vi "Charge Calibration_2011.vi"(0 "Screen&Camera 2":T1={"Screen Orientation"="Regular", "Screen angle"="Flat", "Lens"=enum."FL1-f8x08", "Calibration (mm/pix)"=1.0}, 1 "ROI infos":T3={"npix-X"=512, "npix-Y"=384, "Left [pix]"=0.0, "Top [pix]"=0.0}, 2 "Image (Counts)":dbl[][](array[numeric]), 3 "Filters":cluster{"Name":string, "#Filters":dbl}[](array[cluster])=[{"Name"="BG38", "#Filters"=0.0}, {"Name"="F40", "#Filters"=0.0}, {"Name"="F70", "#Filters"=0.0}, {"Name"="oldBP", "#Filters"=0.0}], 4 "Electron energy (MeV)":dbl=100.0) -> (7 "Image (pC)":dbl[][](array[numeric]))   [LabVIEW 2020]
uses:
  SubVis/ScreenCam2_TypDEf.ctl
  MagAnalysis_Online_Bella/SubVis/CamAndObj_TypDEf.ctl
panel:
  # "Screen Charge calibration\n10/06/10 - Guillaume Plateau"
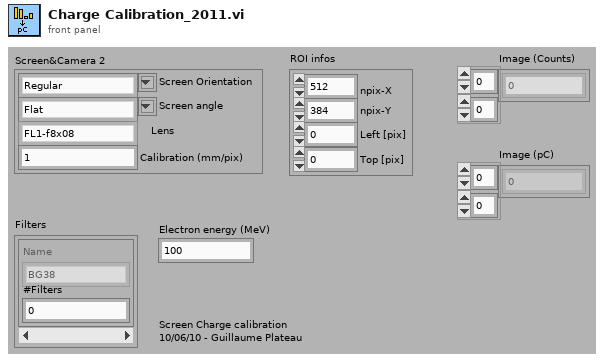
[diagram p1: front panel]
types:
  T1 = typedef "ScreenCam2_TypDEf.ctl" = cluster{"Screen Orientation":string, "Screen angle":string, "Lens":T2, "Calibration (mm/pix)":dbl}
  T2 = typedef "CamAndObj_TypDEf.ctl" = enum16{"FL1-f8x08", "FL1-f8x06", "FL1-f8", "ch300-f50", "FL2G-f8", "FL3M14-f8", "FL3M14-f8x08", "FL3M14-f8x08(2x2)", "aca720-f8", "aca1440-f8"}
  T3 = cluster{"npix-X":i32, "npix-Y":i32, "Left [pix]":dbl, "Top [pix]":dbl}
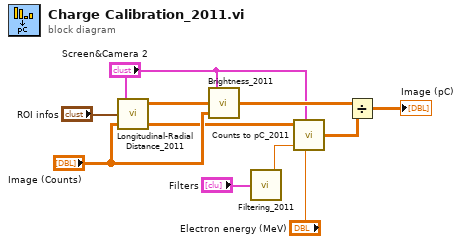
[diagram p0: block diagram]
diagram:
  n1 = call "Longitudinal-Radial Distance_2011.vi"("Image (Counts)"="Image (Counts)", "ROI infos"="ROI infos", "Screen&Camera"="Screen&Camera 2") -> ("Z map"=w7:dbl[][], "R^2 map"=w9:dbl[][])  [unwired: 1 out]
  n2 = call "Brightness_2011.vi"("Image (Counts)"="Image (Counts)", "R^2 map"=w9, "Screen&Camera 2"="Screen&Camera 2") -> ("Corrected image"=w4:dbl[][])  [unwired: 2 out]
  n3 = call "Filtering_2011.vi"("Filters"="Filters") -> ("Filter factor"=w6:dbl)  [unwired: 4 out]
  n4 = call "Counts to pC_2011.vi"("Z map"=w7, "Screen&Camera 2"="Screen&Camera 2", "Filter factor"=w6, "Electron energy (MeV)"="Electron energy (MeV)") -> ("Counts/pC"=w3:dbl[][])  [unwired: 5 out]
  n5 = Divide(x=w4, y=w3) -> (x/y=→"Image (pC)":dbl[][])
